vi "Find.vi"(8 "error in (no error)":errorcluster, 11 "component objects":refnum<class>[](array[class])) -> (0 "error out":errorcluster, 2 "found?":bool, 3 "Transceiver":refnum<class "Transceiver.lvclass">)   [LabVIEW 2017, in "DSF Core.lvlib" / "Transceiver.lvclass"]
uses:
  Transceiver.lvclass
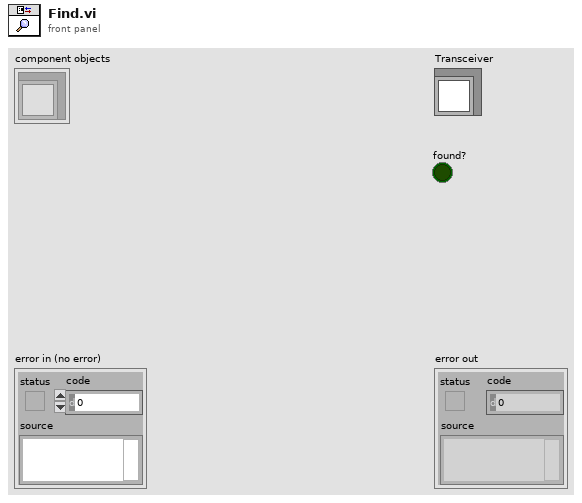
[diagram p1: front panel]
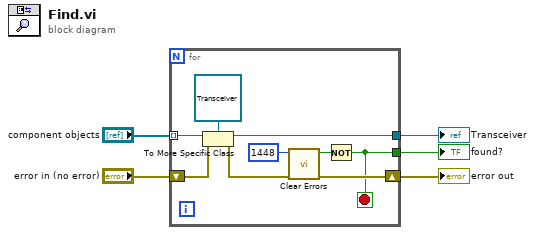
[diagram p0: block diagram]
diagram:
  n1 = for {
    tunnel: "component objects" -> [w13] mode=indexing
    tunnel: [w12] -> w2
    shift-right: [w9] -> w3
    shift-left: "error in (no error)" -> [w8]
    tunnel: [w6] -> w1
    stop <- w6 stop-if-true
    n2 = To More Specific Class(target class=refnum<class "Transceiver.lvclass"> refnum ("DSF.Engine.lvlib:Transceiver"), reference=w13, error in=w8) -> (specific class reference=w12:refnum<class "Transceiver.lvclass">, error out=w10:errorcluster)
    n3 = call <vilib>:"Clear Errors.vi"("error in (no error)"=w10, "specific error code to clear (0: all)"=1448) -> ("error out"=w9:errorcluster, "specific error cleared?"=w7:bool)  [unwired: 4 in]
    n4 = Not(x=w7) -> (.not. x?=w6:bool)
  }
  "error out" <- w3
  "Transceiver" <- w2
  "found?" <- w1
